vi "Check Includes Coordinate.vi"(8 "Error In":errorcluster, 10 "Coordinate":T1, 11 "Panel Object in":refnum<class "Panel Object.lvclass">) -> (0 "Error Out":errorcluster, 2 "Included?":bool, 3 "Panel Object out":refnum<class "Panel Object.lvclass">)   [LabVIEW 2015, in "Panel Object.lvclass"]
uses:
  Panel Object.lvclass
  Typedefs/Point--Cluster.ctl
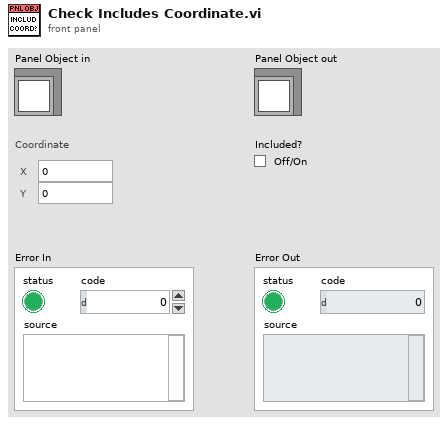
[diagram p1: front panel]
types:
  T1 = typedef "Point--Cluster.ctl" = cluster{"Horizontal":i32, "Vertical":i32}
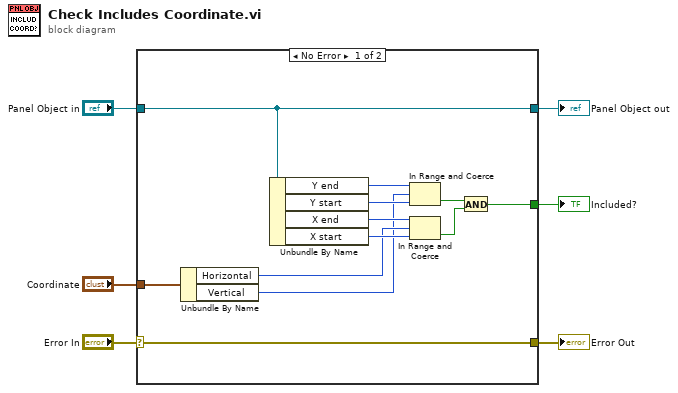
[diagram p0: block diagram]
diagram:
  n1 = case shown="No Error" "Error In" {
    selector: "Error In" -> [w18 w20]
    tunnel: [w18 w20] -> w3
    tunnel: [w11 w19] -> w5
    tunnel: "Panel Object in" -> [w11 w19]
    tunnel: [w10 _] -> w2
    tunnel: "Coordinate" -> [w9 _]
    frame No Error {
      n2 = Unbundle By Name(w9) -> ("Horizontal"=w8:i32, "Vertical"=w7:i32)
      n3 = Unbundle By Name(w11) -> ("Y end"=w17:i32, "Y start"=w16:i32, "X end"=w15:i32, "X start"=w14:i32)
      n4 = In Range and Coerce(upper limit=w17, x=w7, lower limit=w16) -> (In Range?=w13:bool)  [unwired: 1 out]
      n5 = In Range and Coerce(upper limit=w15, x=w8, lower limit=w14) -> (In Range?=w12:bool)  [unwired: 1 out]
      n6 = And(x=w13, y=w12) -> (x .and. y?=w10:bool)
    }
    frame Error {
    }
  }
  "Panel Object out" <- w5
  "Error Out" <- w3
  "Included?" <- w2
